vi "dynamic.vi"(8 "error in (no error)":errorcluster, 11 "Child in":refnum<class "Child.lvclass">) -> (0 "error out":errorcluster, 2 "message":string="Parent Dynamic VI", 3 "Child out":refnum<class "Child.lvclass">)   [LabVIEW 2024, in "Child.lvclass"]
uses:
  Child.lvclass
  Parent/Parent.lvclass
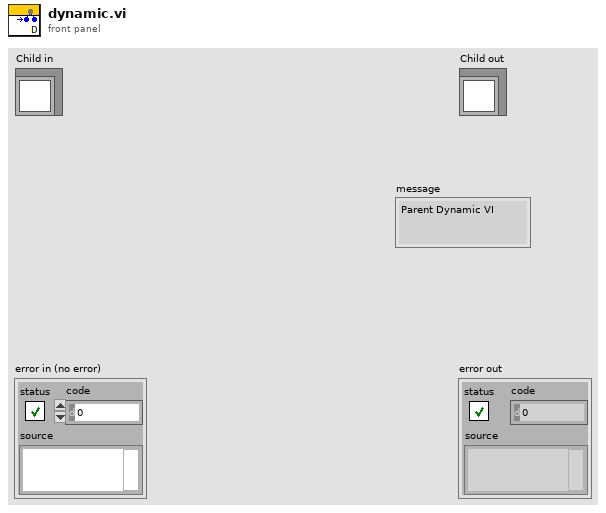
[diagram p1: front panel]
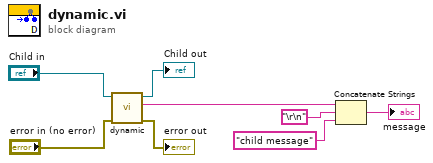
[diagram p0: block diagram]
diagram:
  n1 = call-parent "dynamic.vi"("error in (no error)"="error in (no error)", "parent in"="Child in") -> ("error out"=→"error out":errorcluster, "message"=w4:string, "parent out"=→"Child out":refnum<class "Child.lvclass">)  [unwired: 7 in]
  n2 = Concatenate Strings(w4, "\r\n", "child message" ("string")) -> (→"message":string)
